vi "Random Name Generator.vi"() -> (3 "Name":string)   [LabVIEW 2020]
doc: "Returns a random name from a name file."
uses:
  <vilib>/Utility/file.llb/Read Delimited Spreadsheet (string).vi
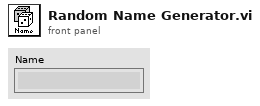
[diagram p1: front panel]
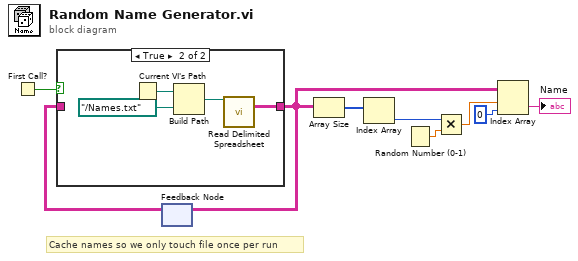
[diagram p0: block diagram]
diagram:
  # "Cache names so we only touch file once per run"
  n1 = First Call?() -> (First Call?: T/F=w3:bool)
  n2 = feedback #1() -> (w2:string[][])  [unwired: 1 in]
  n3 = case shown="True" w3 {
    tunnel: [w10 w11] -> w1
    tunnel: w2 -> [w10 _]
    frame False {
    }
    frame True {
      n4 = Current VI's Path() -> (path=w12:path)
      n5 = Build Path(base path=w12, name or relative path=path "../Names.txt") -> (appended path=w14:path)
      n6 = call-poly <vilib>:"Read Delimited Spreadsheet.vi"("file path (dialog if empty)"=w14) -> ("all rows"=w11:string[][])  [unwired: 9 in, 5 out]
    }
  }
  n7 = feedback-in #1(w1) -> ()
  n8 = Array Size(array=w1) -> (size(s)=w8:i32[])
  n9 = Index Array(array=w8) -> (element=w7:i32)  [unwired: 1 in]
  n10 = Random Number (0-1)() -> (number: 0 to 1=w9:dbl)
  n11 = Multiply(x=w7, y=w9) -> (x*y=w6:dbl)
  n12 = Index Array(array=w1, index (row)=w6, index (col)=0 ("disabled index (col)")) -> (element=→"Name":string)
